vi "Trayectoria.vi"() -> ()   [LabVIEW 2016]
panel:
  in  "CAPTURAR":bool
  in  "DETENER":bool
  in  "BORRAR":bool
  in  "Longitud":dbl(slide) scale=-180.0..180.0
  in  "Latitud":dbl(slide) scale=-90.0..90.0
  out "Trayectoria":cluster{dbl[], dbl[]}(graph)
  out "Posicion":cluster{dbl[], dbl[]}(graph)
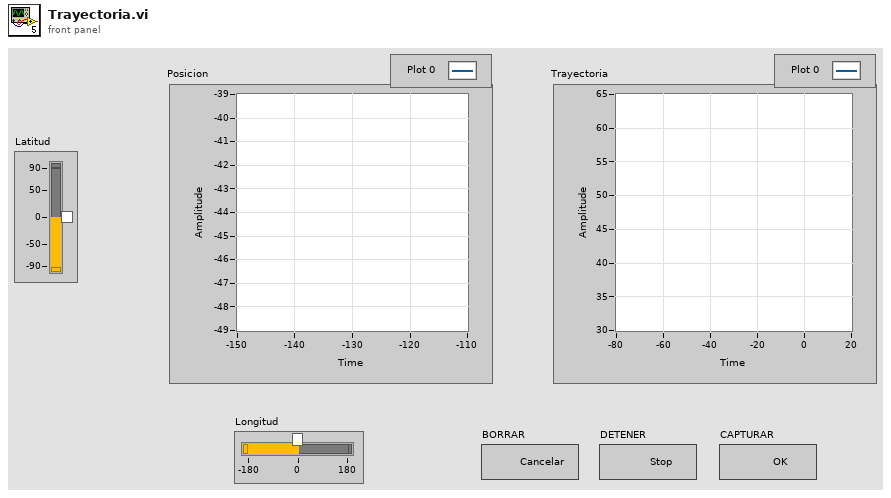
[diagram p1: front panel]
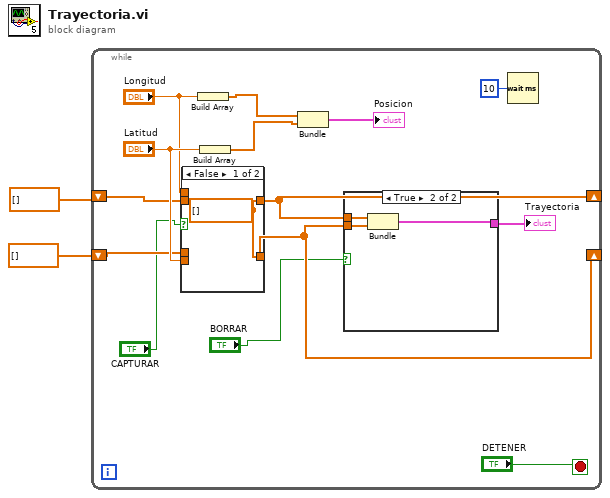
[diagram p0: block diagram]
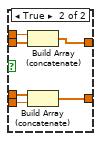
[diagram p3: hidden frame]
diagram:
  n1 = while {
    shift-right: [w10] -> _
    shift-left: dbl[] [] ("Array") -> [w12]
    shift-right: [w9] -> _
    shift-left: dbl[] [] ("Array") -> [w11]
    stop <- "DETENER" stop-if-true
    n2 = case shown="False" "CAPTURAR" {
      tunnel: "Latitud" -> [_ w26]
      tunnel: "Longitud" -> [_ w25]
      tunnel: w12 -> [_ w24]
      tunnel: w11 -> [_ w23]
      tunnel: [w20 w22] -> w10
      tunnel: [w20 w21] -> w9
      frame False {
        w20 = dbl[] [] ("Array")
      }
      frame True {
        n3 = Build Array (concatenate)(w25, w24) -> (w22:dbl[])
        n4 = Build Array (concatenate)(w23, w26) -> (w21:dbl[])
      }
    }
    n5 = Build Array("Longitud") -> (w8:dbl[])
    n6 = Build Array("Latitud") -> (w7:dbl[])
    n7 = Bundle(w8, w7) -> (→"Posicion":cluster{dbl[], dbl[]})  [unwired: 1 in]
    n8 = case shown="True" "BORRAR" {
      tunnel: w10 -> [_ w19]
      tunnel: w9 -> [_ w18]
      tunnel: [_ w17] -> w3
      frame False {
      }
      frame True {
        n9 = Bundle("Array"=w19, "Array"=w18) -> (w17:cluster{"Array":dbl[], "Array":dbl[]})  [unwired: 1 in]
      }
    }
    "Trayectoria" <- w3
    n10 = Wait (ms)(milliseconds to wait=u32 10) -> ()  [unwired: 1 out]
  }
